vi "destroy.vi"(0 "agent_simple_qa in":refnum<class "agent_simple_qa.lvclass">, 11 "error in (no error)":errorcluster) -> (4 "agent_simple_qa out":refnum<class "agent_simple_qa.lvclass">, 15 "error out":errorcluster)   [LabVIEW 2020, in "agent_simple_qa.lvclass"]
uses:
  agent_simple_qa.lvclass
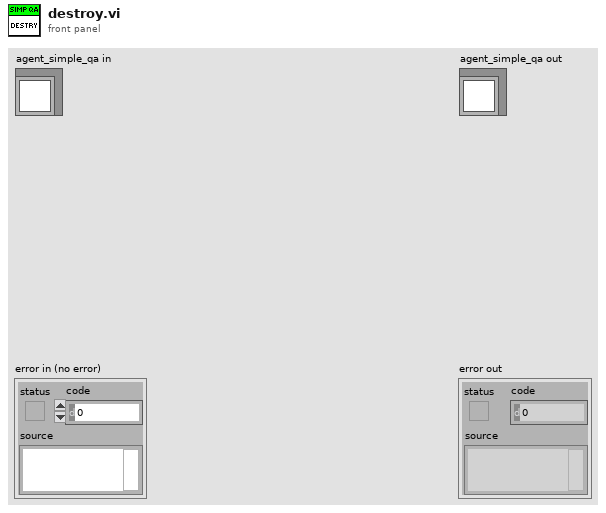
[diagram p1: front panel]
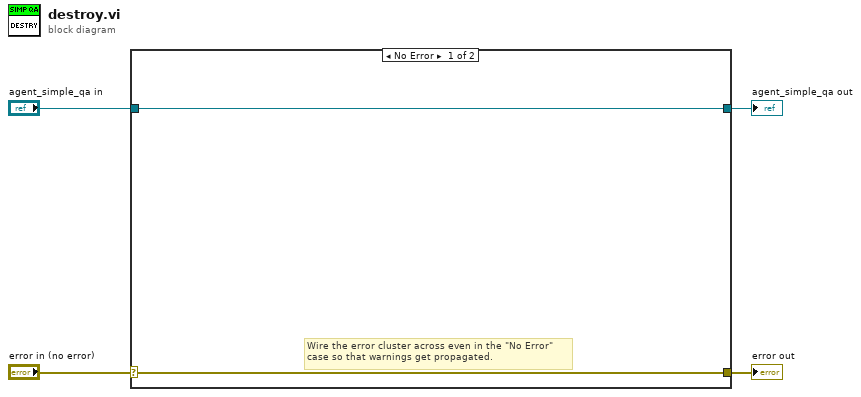
[diagram p0: block diagram]
diagram:
  n1 = case shown="No Error" "error in (no error)" {
    selector: "error in (no error)" -> [w5 w8]
    tunnel: [w5 w8] -> w3
    tunnel: [w6 w7] -> w1
    tunnel: "agent_simple_qa in" -> [w6 w7]
    frame No Error {
      # "Wire the error cluster across even in the \"No Error\"\ncase so that warnings get propagated."
    }
    frame Error {
    }
  }
  "error out" <- w3
  "agent_simple_qa out" <- w1
